vi "CreateDualAxisEncoderTask.vi"(7 "InitialPosition":dbl[](array[numeric]), 8 "error in":errorcluster, 10 "number of samples":i32=1000) -> (0 "error out":errorcluster, 2 "task out (Y)":refnum<k21> caption="task out", 3 "task out (X)":refnum<k21> caption="task out")   [LabVIEW 2014, in "EncoderReadout(NI-DAQmx).lvlib"]
uses:
  EncoderReadout(NI-DAQmx).lvlib
  <vilib>/DAQmx/create/channels.llb/DAQmx Create Channel (CI-Position-Linear Encoder).vi
  <vilib>/DAQmx/configure/timing.llb/DAQmx Timing (Sample Clock).vi
  <resource>/objmgr/daqmx.rc
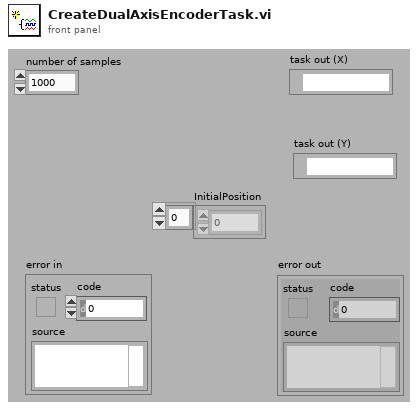
[diagram p1: front panel]
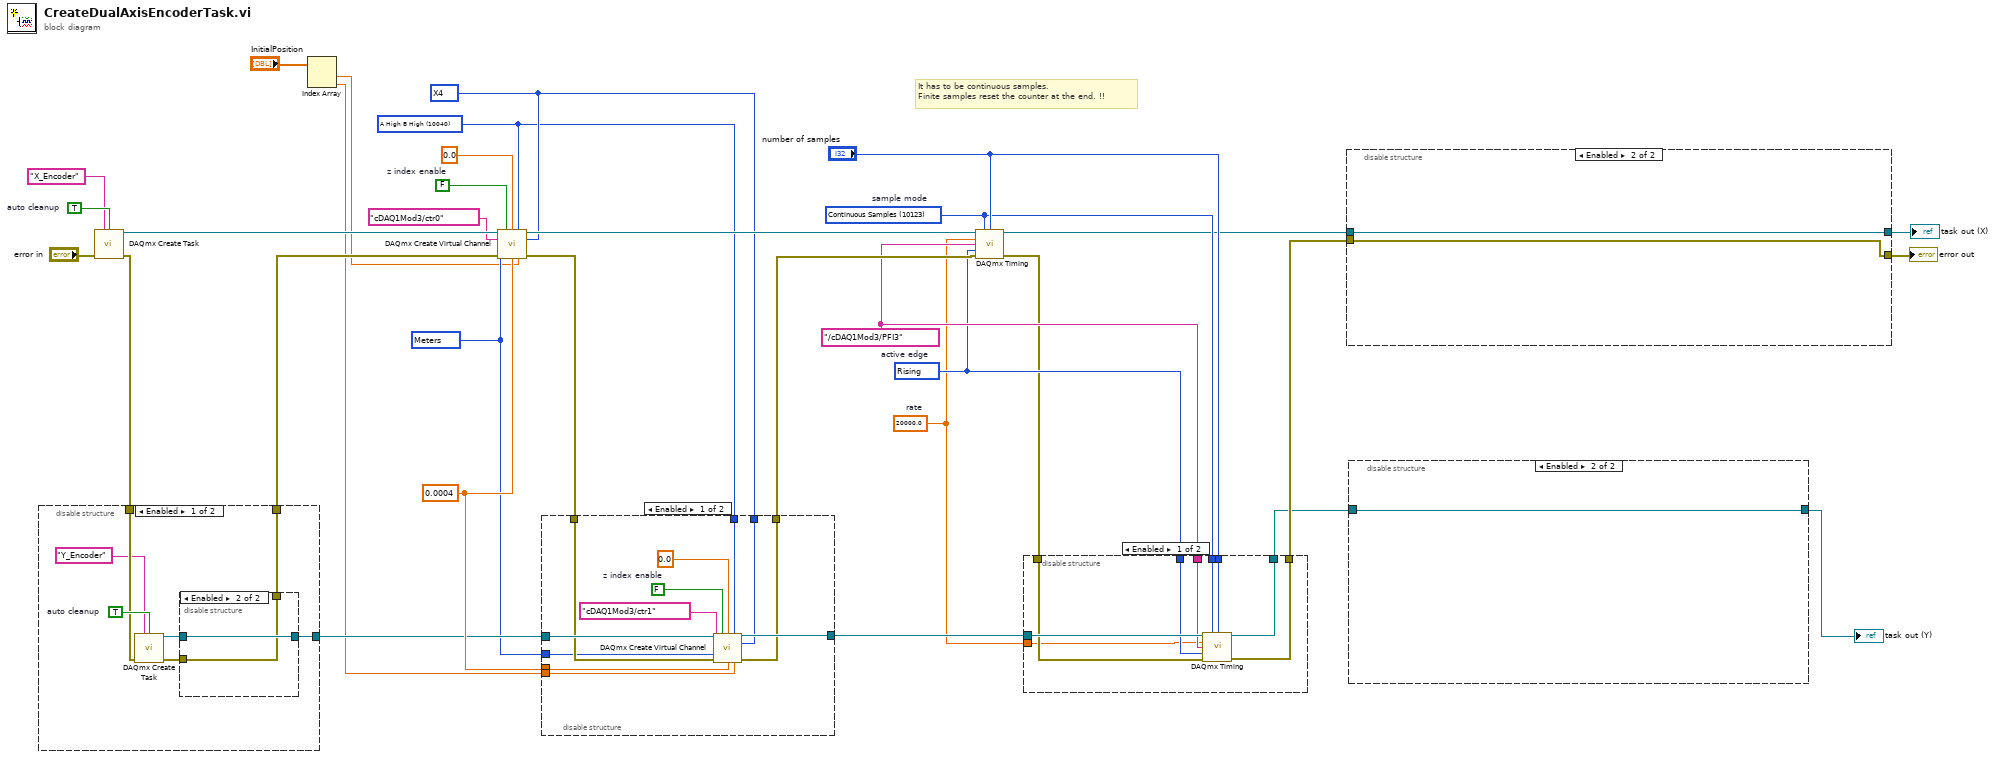
[diagram p0: block diagram]
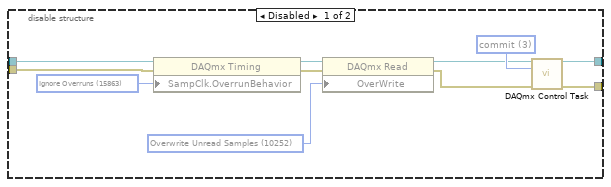
[diagram p2: hidden frame]
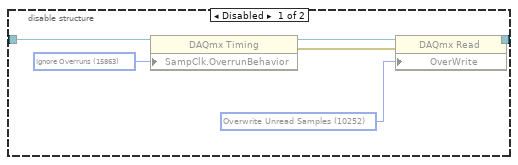
[diagram p3: hidden frame]
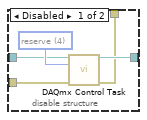
[diagram p4: hidden frame]
diagram:
  w17 = tag "/cDAQ1Mod3/PFI3" ("source")
  w15 = 10123 items=["Finite Samples"=10178, "Continuous Samples"=10123, "Hardware Timed Single Point"=12522]  # sample mode
  w9 = 20000.0  # rate
  w16 = 10280 items=["Rising"=10280, "Falling"=10171]  # active edge
  w6 = 10219 items=["Meters"=10219, "Inches"=10379, "Ticks"=10304, "From Custom Scale"=10065] ("units")
  w8 = 10092 items=["X1"=10090, "X2"=10091, "X4"=10092, "Two Pulse Counting"=10313] ("decoding type")
  w24 = 0.0004 ("distance per pulse")
  w7 = 10040 items=["A High B High"=10040, "A High B Low"=10041, "A Low B High"=10042, "A Low B Low"=10043] ("z index phase")
  w30 = FALSE  # z index enable
  w32 = TRUE  # auto cleanup
  # "It has to be continuous samples. \nFinite samples reset the counter at the end. !!"
  n1 = call <vilib>:"DAQmx Create Task.vi"("new task name"="X_Encoder", "auto cleanup"=w32, "error in"="error in") -> ("task out"=w31:refnum<k21>, "error out"=w22:errorcluster)  [unwired: 11 in]
  n2 = disable-structure shown="Enabled" {
    disable-tunnel: [w34 w48] -> w23
    disable-tunnel: w22 -> [w39 w48]
    disable-tunnel: [w37 _] -> w20
    frame Enabled {
      w40 = TRUE  # auto cleanup
      n3 = call <vilib>:"DAQmx Create Task.vi"("new task name"="Y_Encoder", "auto cleanup"=w40, "error in"=w39) -> ("task out"=w36:refnum<k21>, "error out"=w35:errorcluster)  [unwired: 11 in]
      n4 = disable-structure shown="Enabled" {
        disable-tunnel: [w44 w47] -> w37
        disable-tunnel: w36 -> [w43 w47]
        disable-tunnel: w35 -> [w42 w46]
        disable-tunnel: [w41 w46] -> w34
        frame Disabled {
          w45 = 4 items=["verify"=2, "reserve"=4, "commit"=3, "unreserve"=5, "abort"=6] ("action")
          n5 = call <vilib>:"DAQmx Control Task.vi"("task/channels in"=w43, "action"=w45, "error in"=w42) -> ("task out"=w44:refnum<k21>, "error out"=w41:errorcluster)  [unwired: 11 in]
        }
        frame Enabled {
        }
      }
    }
    frame Disabled {
    }
  }
  n6 = Index Array(array="InitialPosition") -> (element #1=w4:dbl, element #2=w3:dbl)  [unwired: 2 in]
  n7 = call-poly <vilib>:"DAQmx Create Virtual Channel.vi"("task in"=w31, "z index enable"=w30, "z index value"=0.0, "z index phase"=w7, "counter"=tag "cDAQ1Mod3/ctr0", "decoding type"=w8, "units"=w6, "error in"=w23, "distance per pulse"=w24, "initial position"=w4) -> ("task out"=w28:refnum<k21>, "error out"=w19:errorcluster)  [unwired: 4 in]
  n8 = disable-structure shown="Enabled" {
    disable-tunnel: [w58 w62] -> w27
    disable-tunnel: w24 -> [w56 _]
    disable-tunnel: w20 -> [w55 w62]
    disable-tunnel: w19 -> [w54 w61]
    disable-tunnel: [w53 w61] -> w18
    disable-tunnel: w8 -> [w52 _]
    disable-tunnel: w7 -> [w51 _]
    disable-tunnel: w6 -> [w50 _]
    disable-tunnel: w3 -> [w49 _]
    frame Enabled {
      w60 = FALSE  # z index enable
      n9 = call-poly <vilib>:"DAQmx Create Virtual Channel.vi"("task in"=w55, "z index enable"=w60, "z index value"=0.0, "z index phase"=w51, "counter"=tag "cDAQ1Mod3/ctr1", "decoding type"=w52, "units"=w50, "error in"=w54, "distance per pulse"=w56, "initial position"=w49) -> ("task out"=w58:refnum<k21>, "error out"=w53:errorcluster)  [unwired: 4 in]
    }
    frame Disabled {
    }
  }
  n10 = call-poly <vilib>:"DAQmx Timing.vi"("task/channels in"=w28, "sample mode"=w15, "samples per channel"="number of samples", "rate"=w9, "source"=w17, "active edge"=w16, "error in"=w18) -> ("task out"=w11:refnum<k21>, "error out"=w10:errorcluster)  [unwired: 7 in]
  n11 = disable-structure shown="Enabled" {
    disable-tunnel: w27 -> [w71 w73]
    disable-tunnel: "number of samples" -> [w70 _]
    disable-tunnel: w17 -> [w69 _]
    disable-tunnel: w16 -> [w68 _]
    disable-tunnel: w15 -> [w67 _]
    disable-tunnel: [w66 w72] -> w14
    disable-tunnel: [w65 w73] -> w13
    disable-tunnel: w10 -> [w64 w72]
    disable-tunnel: w9 -> [w63 _]
    frame Enabled {
      n12 = call-poly <vilib>:"DAQmx Timing.vi"("task/channels in"=w71, "sample mode"=w67, "samples per channel"=w70, "rate"=w63, "source"=w69, "active edge"=w68, "error in"=w64) -> ("task out"=w65:refnum<k21>, "error out"=w66:errorcluster)  [unwired: 7 in]
    }
    frame Disabled {
    }
  }
  n13 = disable-structure shown="Enabled" {
    disable-tunnel: w14 -> [w84 w85]
    disable-tunnel: w11 -> [w83 w86]
    disable-tunnel: [w76 w86] -> w2
    disable-tunnel: [w74 w85] -> w1
    frame Disabled {
      w78 = 3 items=["verify"=2, "reserve"=4, "commit"=3, "unreserve"=5, "abort"=6] ("action")
      w81 = 10252 items=["Overwrite Unread Samples"=10252, "Do Not Overwrite Unread Samples"=10159] ("OverWrite")
      w82 = 15863 items=["Stop Task And Error"=15862, "Ignore Overruns"=15863] ("SampClk.OverrunBehavior")
      n14 = property class="DAQmx Timing"(reference=w83, error in=w84, "SampClk.OverrunBehavior"=w82) -> (reference out=w80:refnum<k21>, error out=w79:errorcluster)
      n15 = property class="DAQmx Read"(reference=w80, error in=w79, "OverWrite"=w81) -> (reference out=w77:refnum<k21>, error out=w75:errorcluster)
      n16 = call <vilib>:"DAQmx Control Task.vi"("task/channels in"=w77, "action"=w78, "error in"=w75) -> ("task out"=w76:refnum<k21>, "error out"=w74:errorcluster)  [unwired: 11 in]
    }
    frame Enabled {
    }
  }
  "error out" <- w1
  "task out (X)" <- w2
  n17 = disable-structure shown="Enabled" {
    disable-tunnel: w13 -> [w92 w93]
    disable-tunnel: [w91 w93] -> w12
    frame Disabled {
      w88 = 10252 items=["Overwrite Unread Samples"=10252, "Do Not Overwrite Unread Samples"=10159] ("OverWrite")
      w87 = 15863 items=["Stop Task And Error"=15862, "Ignore Overruns"=15863] ("SampClk.OverrunBehavior")
      n18 = property class="DAQmx Timing"(reference=w92, "SampClk.OverrunBehavior"=w87) -> (reference out=w89:refnum<k21>, error out=w90:errorcluster)  [unwired: 1 in]
      n19 = property class="DAQmx Read"(reference=w89, error in=w90, "OverWrite"=w88) -> (reference out=w91:refnum<k21>)  [unwired: 1 out]
    }
    frame Enabled {
    }
  }
  "task out (Y)" <- w12
